vi "报文记录更新.vi"(0 "MainPage输入":refnum<class "MainPage.lvclass">, 1 "报文信息记录":string[][](array[string])) -> ()   [LabVIEW 2019, in "MainPage.lvlib" / "MainPage.lvclass"]
uses:
  MainPage.lvclass
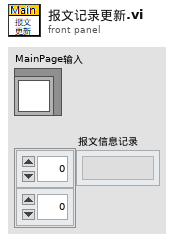
[diagram p1: front panel]
types:
  T1 = typedef "MainPage.lvlib/MainPage.lvclass/DataRef_通讯接口.ctl" = cluster{"连接方式":enum16{"网口(客服端)", "网口(服务端)", "串口"}, "VISA串口名称":refnum<visa-resource-name>, "服务端识别":cluster{"本机IP":string, "本机端口":u16, "当前目标":string, "服务端侦听ID":refnum<k5>}, "客服端识别":cluster{"客P-主IP:Port":string}, "客服端记录":map{string, refnum<k5>}, "服务端接口记录":map{string, refnum<k5>}}
  T2 = cluster{"寄存器模拟":u16[], "串口正常？":bool, "报文信息记录":string[][]}
  T3 = enum16{"ini", "增加记录", "读取记录", "更改寄存器值", "更改接口状态", "更改报文信息", "增加报文信息"}
  T4 = cluster{"串口正常？":bool, "寄存器模拟":u16[], "报文信息记录":string[][]}
  T5 = enum16{"ini", "读取", "写入-报文记录", "写入-寄存器模拟", "写入-串口状态", "增加报文记录"}
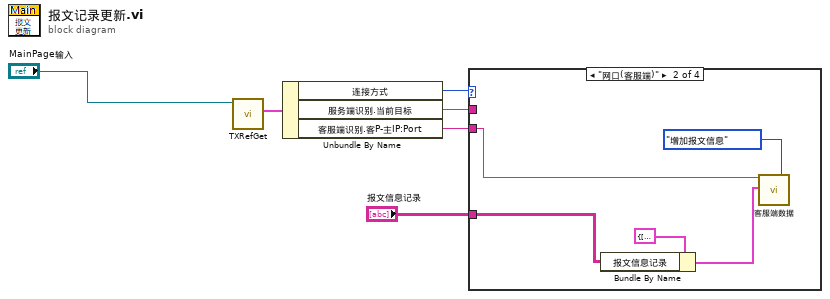
[diagram p0: block diagram]
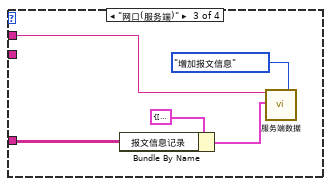
[diagram p3: hidden frame]
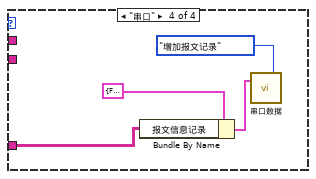
[diagram p4: hidden frame]
diagram:
  n1 = call-dynamic "TXRefGet.vi"("MainPage 输入"="MainPage输入") -> ("通讯接口数据"=w1:T1)  [unwired: 6 in, 4 out]
  n2 = Unbundle By Name(w1) -> ("连接方式"=w6:enum16{"网口(客服端)", "网口(服务端)", "串口"}, "服务端识别.当前目标"=w2:string, "客服端识别.客P-主IP:Port"=w3:string)
  n3 = case shown="\"网口(客服端)\"" w6 {
    tunnel: w2 -> [_ _ w15 _]
    tunnel: w3 -> [_ w10 _ _]
    tunnel: "报文信息记录" -> [_ w8 w13 w18]
    frame Default {
    }
    frame "网口(客服端)" {
      n4 = Bundle By Name(cluster=T2 {"寄存器模拟"=[], "串口正常？"=FALSE, "报文信息记录"=[]} ("数据输入"), "报文信息记录"=w8) -> (w7:T2)
      n5 = call "客服端数据.vi"("客P-主IP:P"=w10, "数据输入"=w7, "枚举"=T3."增加报文信息") -> ()  [unwired: 15 in, 2 out]
    }
    frame "网口(服务端)" {
      n6 = Bundle By Name(cluster=T2 {"寄存器模拟"=[], "串口正常？"=FALSE, "报文信息记录"=[]} ("数据输入"), "报文信息记录"=w13) -> (w12:T2)
      n7 = call "服务端数据.vi"("IP-Port"=w15, "数据输入"=w12, "枚举"=T3."增加报文信息") -> ()  [unwired: 15 in, 2 out]
    }
    frame "串口" {
      n8 = Bundle By Name(cluster=T4 {"串口正常？"=FALSE, "寄存器模拟"=[], "报文信息记录"=[]} ("串口输入"), "报文信息记录"=w18) -> (w17:T4)
      n9 = call "串口数据.vi"("串口输入"=w17, "枚举"=T5."增加报文记录") -> ()  [unwired: 17 in, 1 out]
    }
  }
